vi "Teleop.vi"(10 "Match Info":T1={"Autonomous Elapsed Seconds"=0.0, "TeleOp Elapsed Seconds"=0.0, "Disabled Elapsed Seconds"=0.0, "Visited Autonomous"=FALSE, "Visited TeleOp"=FALSE, "Visited Disabled"=FALSE, "Autonomous Settings"={"Autonomous Style"=enum."Independent", "VI Refnum"=refnum}}, 11 "Call Context":T2) -> ()   [LabVIEW 2020]
doc: "This VI is called for each TeleOp packet received from the DS where the robot is not disabled. It is often used to read from the joysticks and update I/O or to update setpoints for timed control loops. It should complete and return within 20 milliseconds or it may miss DS packets."
uses:
  <vilib>/Rock Robotics/WPI/DriverStation/WPI_DriverStationDerivedRobotMode.ctl
  <vilib>/Rock Robotics/WPI/DriverStation/WPI_DriverStationMatch Info.ctl
  <vilib>/Rock Robotics/WPI/Solenoid/WPI_SolenoidValue.ctl
  <vilib>/Rock Robotics/Network Tables/NT Read Boolean.vi
  <vilib>/Rock Robotics/Network Tables/NT Read Number.vi
  <vilib>/Rock Robotics/WPI/Utilities/WPI_GetSetVariantRefNum.vi
  <vilib>/Rock Robotics/Network Tables/NT Write Numeric Array.vi
  <vilib>/Rock Robotics/WPI/Solenoid/WPI_SolenoidSetEnum.vi
  <vilib>/Rock Robotics/Network Tables/NT Write Boolean Array.vi
  <vilib>/Rock Robotics/WPI/RobotDrive/WPI_RobotDriveArcadeDrive_Standard(NoSaturation).vi
panel:
  out "Sample Slider 0":dbl(slide) scale=0.0..5.0
  out "Sample Boolean 1":bool
  out "Sample Boolean 0":bool
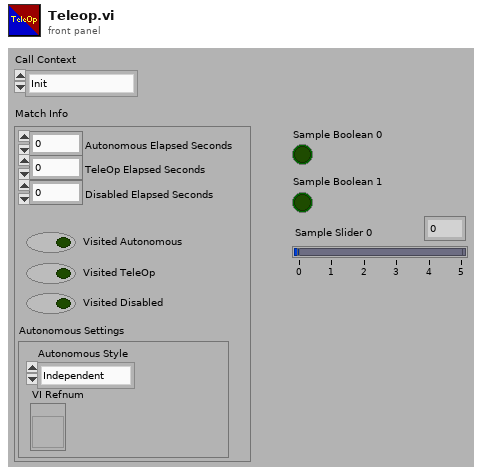
[diagram p1: front panel]
types:
  T1 = typedef "WPI_DriverStationMatch Info.ctl" = cluster{"Autonomous Elapsed Seconds":dbl, "TeleOp Elapsed Seconds":dbl, "Disabled Elapsed Seconds":dbl, "Visited Autonomous":bool, "Visited TeleOp":bool, "Visited Disabled":bool, "Autonomous Settings":cluster{"Autonomous Style":enum16{"Iterative", "Independent"}, "VI Refnum":refnum<vi>}}
  T2 = typedef "WPI_DriverStationDerivedRobotMode.ctl" = enum16{"Init", "Execute", "Stop"}
  T3 = typedef "WPI_SolenoidValue.ctl" = enum16{"Off", "On", "Forward", "Reverse"}
  T4 = typedef "WPI_JoystickDevRef.ctl" = cluster{"Device":T5}
  T5 = typedef "WPI_JoystickDeviceEnum.ctl" = enum16{"USB 0", "USB 1", "USB 2", "USB 3", "USB 4", "USB 5"}
  T6 = cluster{"Axes[0]":dbl, "Axes[1]":dbl, "Axes[2]":dbl, "Axes[3]":dbl, "Axes[4]":dbl, "Axes[5]":dbl, "Axes[6]":dbl, "Axes[7]":dbl, "Axes[8]":dbl}
  T7 = cluster{"Buttons[0]":bool, "Buttons[1]":bool, "Buttons[2]":bool, "Buttons[3]":bool, "Buttons[4]":bool, "Buttons[5]":bool, "Buttons[6]":bool, "Buttons[7]":bool, "Buttons[8]":bool}
  T8 = typedef "WPI_MotorControlDeviceRef.ctl" = cluster{"DeviceStatus":errorcluster, "Type":T9, "PWM":cluster{"PWM Channel":T10, "DeadBand":T11}, "CAN":cluster{"Device Number":u8, "SetOutput VI Ref":variant, "GetOutput VI Ref":variant, "Enable VI Ref":variant, "Disable VI Ref":variant, "Data":variant}, "Invert":bool, "DIO PWM":cluster{"PWM \"Enable\" Channel":T10, "DIOChannel":T12, "PWM Rate":dbl}}
  T9 = typedef "WPI_MotorControlType.ctl" = enum16{"PWM", "CAN", "DIO PWM"}
  T10 = typedef "FPGA_DIOPWMChannel.ctl" = enum8{"PWM 0", "PWM 1", "PWM 2", "PWM 3", "PWM 4", "PWM 5", "PWM 6", "PWM 7", "PWM 8", "PWM 9", "PWM MXP 0", "PWM MXP 1", "PWM MXP 2", "PWM MXP 3", "PWM MXP 4", "PWM MXP 5", "PWM MXP 6", "PWM MXP 7", "PWM MXP 8", "PWM MXP 9", "Invalid"}
  T11 = typedef "WPI_PWMDeadband.ctl" = cluster{"Name":string, "maxPositivePwm":i32, "minPositivePwm":i32, "centerPwm":i32, "maxNegativePwm":i32, "minNegativePwm":i32, "angularRange":u16}
  T12 = typedef "FPGA_DIOChannel.ctl" = enum8{"DIO 0", "DIO 1", "DIO 2", "DIO 3", "DIO 4", "DIO 5", "DIO 6", "DIO 7", "DIO 8", "DIO 9", "DIO MXP 0", "DIO MXP 1", "DIO MXP 2", "DIO MXP 3", "DIO MXP 4", "DIO MXP 5", "DIO MXP 6", "DIO MXP 7", "DIO MXP 8", "DIO MXP 9", "DIO MXP 10", "DIO MXP 11", "DIO MXP 12", "DIO MXP 13", "DIO MXP 14", "DIO MXP 15", "SPI Port CS1", "SPI Port CS2", "SPI Port CS3", "SPI Port MISO", "SPI Port MOSI", "Invalid"}
  T13 = typedef "WPI_SolenoidDevRef.ctl" = cluster{"DevStatus":errorcluster, "Pneumatics Control Module":u8, "Forward Solenoid Channel":T14, "Reverse Solenoid Channel":T14}
  T14 = typedef "WPI_SolenoidChannel.ctl" = enum8{"Solenoid 0", "Solenoid 1", "Solenoid 2", "Solenoid 3", "Solenoid 4", "Solenoid 5", "Solenoid 6", "Solenoid 7", "Solenoid 8", "Solenoid 9", "Solenoid 10", "Solenoid 11", "Solenoid 12", "Solenoid 13", "Solenoid 14", "Solenoid 15", "Invalid"}
  T15 = typedef "WPI_RobotDriveDevRef.ctl" = cluster{"DevStatus":errorcluster, "Motors[]":T8[], "Square Inputs":bool, "Max Output":dbl}
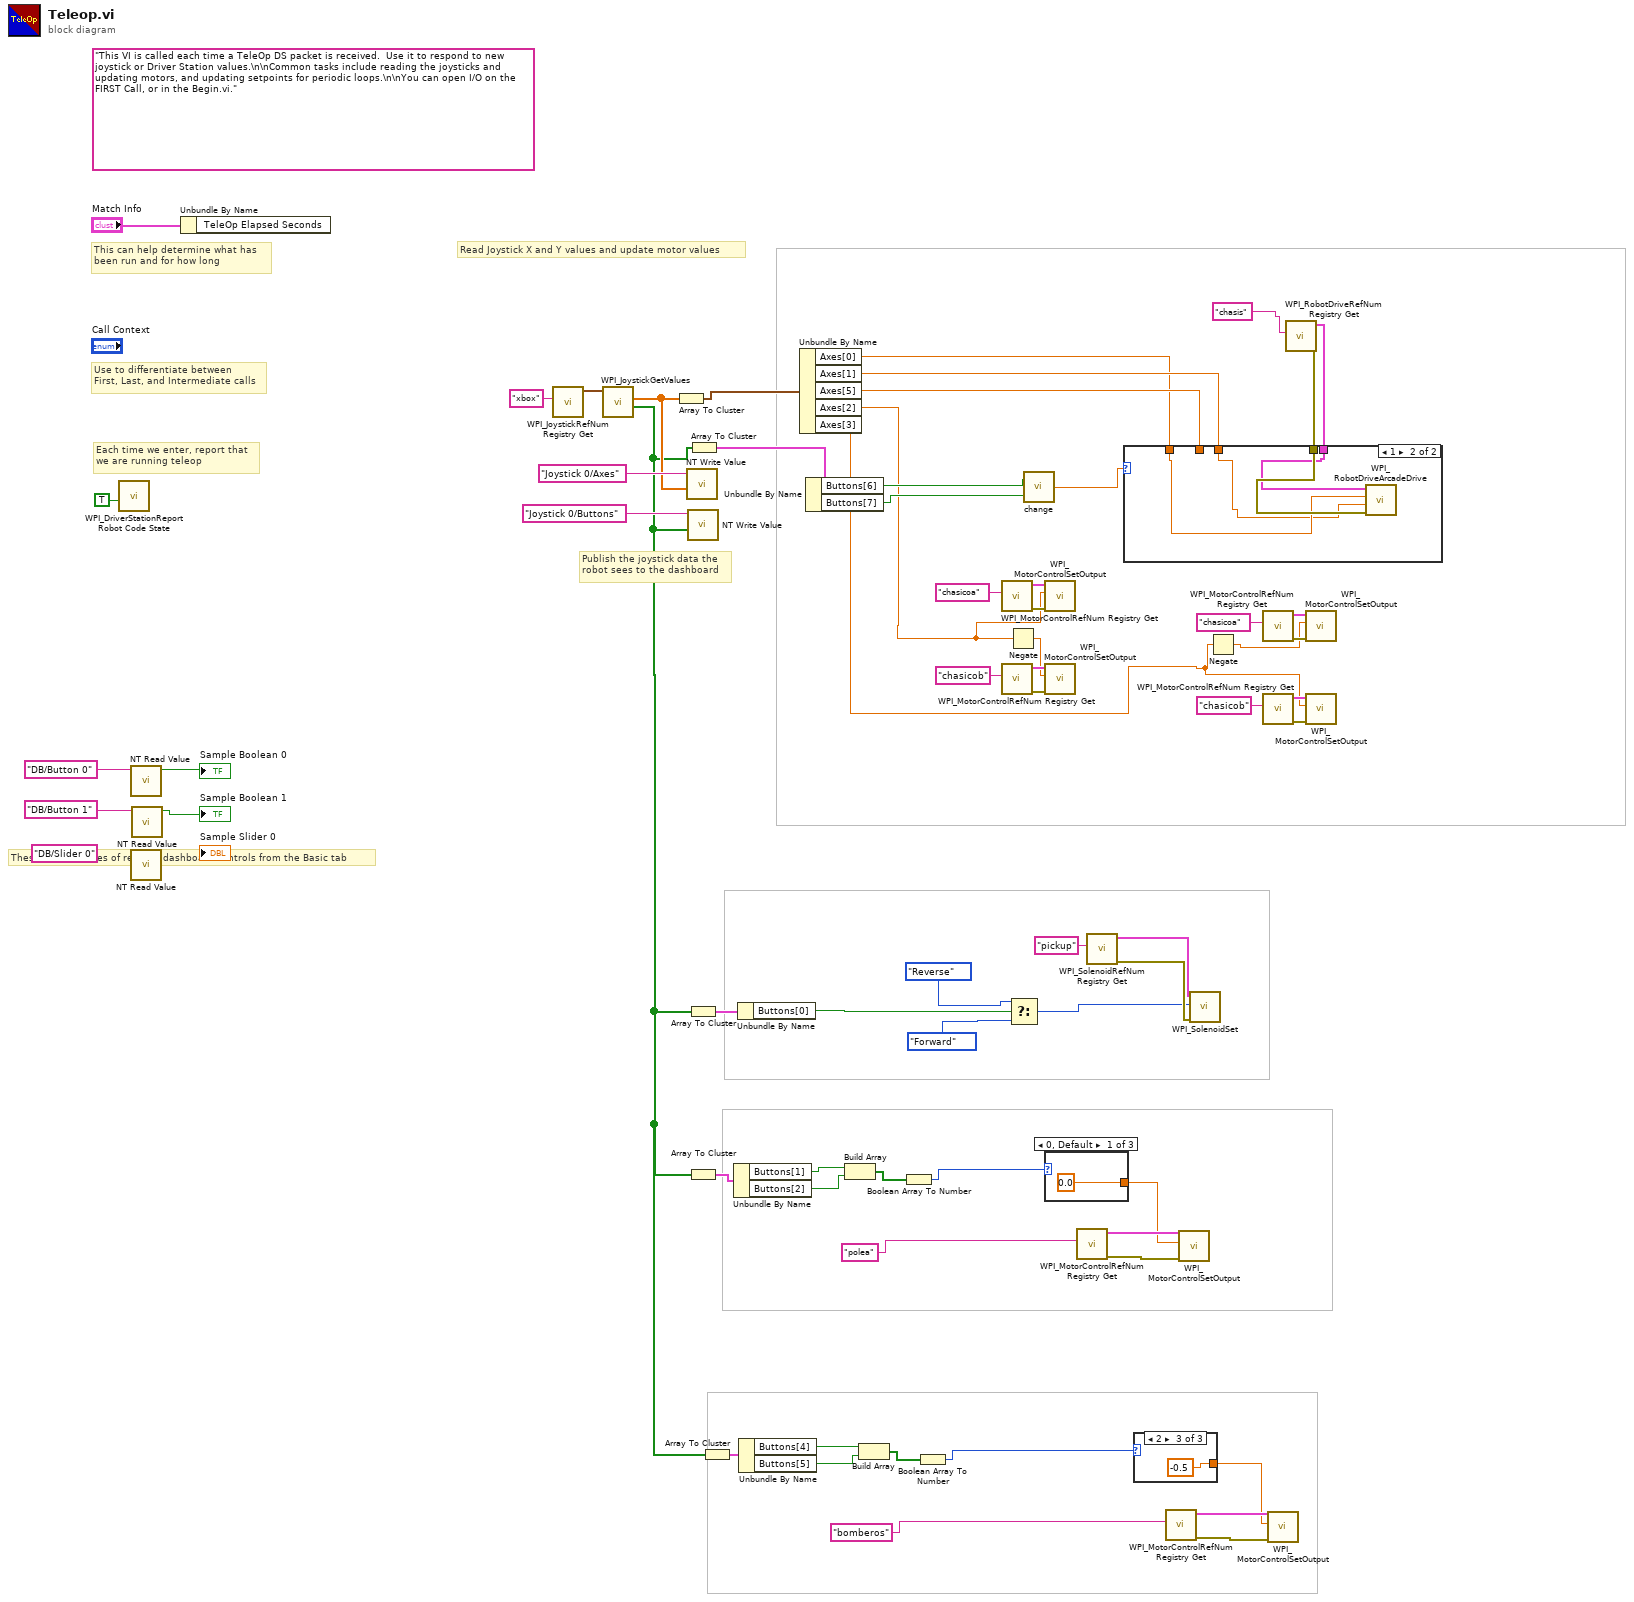
[diagram p0: block diagram]
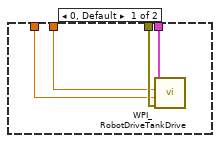
[diagram p2: hidden frame]
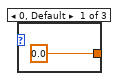
[diagram p3: hidden frame]
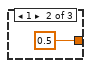
[diagram p4: hidden frame]
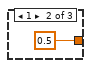
[diagram p5: hidden frame]
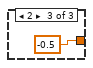
[diagram p6: hidden frame]
diagram:
  (unwired) "This VI is called each time a TeleOp DS packet is received.  Use it to respond to new joystick or Driver Station values.\n\nCommon tasks include reading the joysticks and updating motors, and updating setpoints for periodic loops.\n\nYou can open I/O on the FIRST Call, or in the Begin.vi."
  # "These are examples of reading dashboard controls from the Basic tab"
  # "Publish the joystick data the\nrobot sees to the dashboard"
  # "Each time we enter, report that\nwe are running teleop"
  # "Use to differentiate between\nFirst, Last, and Intermediate calls"
  # "This can help determine what has\nbeen run and for how long"
  # "Read Joystick X and Y values and update motor values"
  n1 = call <vilib>:"WPI_DriverStationReport Robot Code State.vi"("TeleOp"=TRUE ("Autonomous")) -> ()  [unwired: 10 in, 1 out]
  n2 = call-poly <vilib>:"NT Read Value.vi"("Name"="DB/Button 0" ("refnum name")) -> ("Boolean"=→"Sample Boolean 0":bool)  [unwired: 9 in, 1 out]
  n3 = call-poly <vilib>:"NT Read Value.vi"("Name"="DB/Slider 0" ("refnum name")) -> ("Numeric"=→"Sample Slider 0":dbl)  [unwired: 9 in, 1 out]
  n4 = call-poly <vilib>:"NT Read Value.vi"("Name"="DB/Button 1" ("refnum name")) -> ("Boolean"=→"Sample Boolean 1":bool)  [unwired: 9 in, 1 out]
  n5 = Unbundle By Name("Match Info") -> ()  [unwired: 1 out]
  n6 = call <vilib>:"WPI_JoystickRefNum Registry Get.vi"("refnum name"="xbox") -> ("JoystickDevRef"=w66:T4)  [unwired: 1 in, 9 out]
  n7 = call <vilib>:"WPI_JoystickGetValues.vi"("JoystickDevRef"=w66) -> ("Buttons"=w22:bool[], "Axes"=w31:dbl[])  [unwired: 6 in, 3 out]
  n8 = Array To Cluster(array=w31) -> (cluster=w30:T6)
  n9 = call-poly <vilib>:"NT Write Value.vi"("Numeric Array"=w31, "Name"="Joystick 0/Axes") -> ()  [unwired: 9 in, 1 out]
  n10 = call-poly <vilib>:"NT Write Value.vi"("Boolean Array"=w22, "Name"="Joystick 0/Buttons") -> ()  [unwired: 9 in, 1 out]
  n11 = Array To Cluster(array=w22) -> (cluster=w56:T7)
  n12 = Array To Cluster(array=w22) -> (cluster=w48:T7)
  n13 = Array To Cluster(array=w22) -> (cluster=w21:T7)
  n14 = Array To Cluster(array=w22) -> (cluster=w41:T7)
  n15 = Unbundle By Name(w48) -> ("Buttons[1]"=w44:bool, "Buttons[2]"=w43:bool)
  n16 = Unbundle By Name(w56) -> ("Buttons[0]"=w49:bool)
  n17 = Unbundle By Name(w41) -> ("Buttons[4]"=w37:bool, "Buttons[5]"=w36:bool)
  n18 = Unbundle By Name(w30) -> ("Axes[0]"=w12:dbl, "Axes[1]"=w14:dbl, "Axes[5]"=w15:dbl, "Axes[2]"=w10:dbl, "Axes[3]"=w1:dbl)
  n19 = Unbundle By Name(w21) -> ("Buttons[6]"=w20:bool, "Buttons[7]"=w19:bool)
  n20 = Build Array(w44, w43) -> (w32:bool[])
  n21 = Build Array(w37, w36) -> (w35:bool[])
  n22 = Boolean Array To Number(Boolean array=w32) -> (number=w9:u32)
  n23 = Boolean Array To Number(Boolean array=w35) -> (number=w34:u32)
  n24 = call <vilib>:"WPI_MotorControlRefNum Registry Get.vi"("refnum name"="chasicoa") -> ("error out"=w27:errorcluster, "MotorControlDevRef"=w26:T8)  [unwired: 9 in]
  n25 = call <vilib>:"WPI_MotorControlRefNum Registry Get.vi"("refnum name"="chasicob") -> ("error out"=w24:errorcluster, "MotorControlDevRef"=w18:T8)  [unwired: 9 in]
  n26 = Negate(x=w10) -> (-x=w11:dbl)
  n27 = Select(t=WPI_SolenoidValue."Reverse" ("Value"), s=w49, f=WPI_SolenoidValue."Forward" ("Value")) -> (s? t:f=w51:T3)
  n28 = call "change.vi"("start"=w19, "back"=w20) -> ("output"=w17:dbl)
  n29 = call <vilib>:"WPI_MotorControlSetOutput.vi"("error in (no error)"=w27, "Output"=w10, "MotorControlDevRef"=w26) -> ()  [unwired: 6 in, 3 out]
  n30 = call <vilib>:"WPI_MotorControlSetOutput.vi"("error in (no error)"=w24, "Output"=w11, "MotorControlDevRef"=w18) -> ()  [unwired: 6 in, 3 out]
  n31 = case shown="0, Default" w9 {
    tunnel: [0.0 0.5 -0.5] -> w42
    frame 0, Default {
    }
    frame 1 {
    }
    frame 2 {
    }
  }
  n32 = call <vilib>:"WPI_MotorControlRefNum Registry Get.vi"("refnum name"="polea") -> ("error out"=w45:errorcluster, "MotorControlDevRef"=w46:T8)  [unwired: 9 in]
  n33 = call <vilib>:"WPI_SolenoidRefNum Registry Get.vi"("refnum name"="pickup") -> ("error out"=w54:errorcluster, "SolenoidDevRef"=w55:T13)  [unwired: 9 in]
  n34 = case shown="2" w34 {
    tunnel: [0.0 0.5 -0.5] -> w33
    frame 0, Default {
    }
    frame 1 {
    }
    frame 2 {
    }
  }
  n35 = call <vilib>:"WPI_MotorControlRefNum Registry Get.vi"("refnum name"="bomberos") -> ("error out"=w38:errorcluster, "MotorControlDevRef"=w39:T8)  [unwired: 9 in]
  n36 = call <vilib>:"WPI_MotorControlSetOutput.vi"("error in (no error)"=w45, "Output"=w42, "MotorControlDevRef"=w46) -> ()  [unwired: 6 in, 3 out]
  n37 = call-poly <vilib>:"WPI_SolenoidSet.vi"("error in (no error)"=w54, "Value"=w51, "SolenoidDevRef"=w55) -> ()  [unwired: 7 in, 2 out]
  n38 = Negate(x=w1) -> (-x=w2:dbl)
  n39 = call <vilib>:"WPI_MotorControlRefNum Registry Get.vi"("refnum name"="chasicoa") -> ("error out"=w8:errorcluster, "MotorControlDevRef"=w7:T8)  [unwired: 9 in]
  n40 = call <vilib>:"WPI_MotorControlRefNum Registry Get.vi"("refnum name"="chasicob") -> ("error out"=w5:errorcluster, "MotorControlDevRef"=w3:T8)  [unwired: 9 in]
  n41 = call <vilib>:"WPI_MotorControlSetOutput.vi"("error in (no error)"=w38, "Output"=w33, "MotorControlDevRef"=w39) -> ()  [unwired: 6 in, 3 out]
  n42 = call <vilib>:"WPI_RobotDriveRefNum Registry Get.vi"("refnum name"="chasis") -> ("error out"=w16:errorcluster, "RobotDriveDevRef"=w13:T15)  [unwired: 9 in]
  n43 = case shown="1" w17 {
    tunnel: w16 -> [w77 w81]
    tunnel: w15 -> [w74 _]
    tunnel: w14 -> [w75 w79]
    tunnel: w13 -> [w76 w78]
    tunnel: w12 -> [_ w80]
    frame 0, Default {
      n44 = call <vilib>:"WPI_RobotDriveTankDrive.vi"("error in (no error)"=w77, "Right axis value"=w74, "Left axis value"=w75, "RobotDriveDevRef"=w76) -> ()  [unwired: 5 in, 3 out]
    }
    frame 1 {
      n45 = call-poly <vilib>:"WPI_RobotDriveArcadeDrive.vi"("error in (no error)"=w81, "Y axis value"=w79, "X axis value"=w80, "RobotDriveDevRef"=w78) -> ()  [unwired: 5 in, 3 out]
    }
  }
  n46 = call <vilib>:"WPI_MotorControlSetOutput.vi"("error in (no error)"=w8, "Output"=w2, "MotorControlDevRef"=w7) -> ()  [unwired: 6 in, 3 out]
  n47 = call <vilib>:"WPI_MotorControlSetOutput.vi"("error in (no error)"=w5, "Output"=w1, "MotorControlDevRef"=w3) -> ()  [unwired: 6 in, 3 out]
